vi "serialWrite.vi"(8 "error in (no error)":errorcluster, 10 "text":string, 11 "Python":T1) -> (0 "error out":errorcluster, 3 "Num loops":i32)   [LabVIEW 2020]
uses:
  PythonCtrl.ctl
  Processors.ctl
panel:
  out "appended array":i32[](array[numeric])
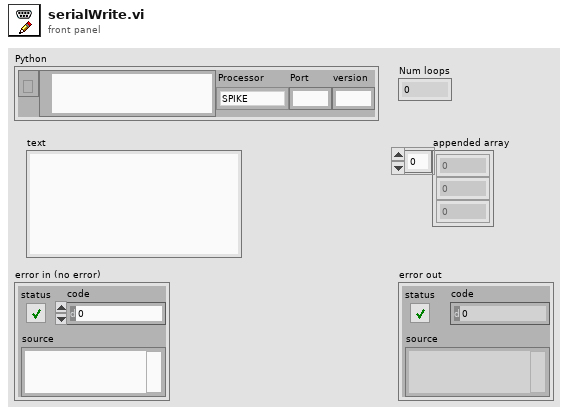
[diagram p1: front panel]
types:
  T1 = typedef "PythonCtrl.ctl" = cluster{"session":refnum<k35>, "PyPath":path, "Processor":T2, "Port":string, "version":string}
  T2 = typedef "Processors.ctl" = enum16{"SPIKE", "Pi", "Pi_ssh", "OpenMV", "Dunio"}
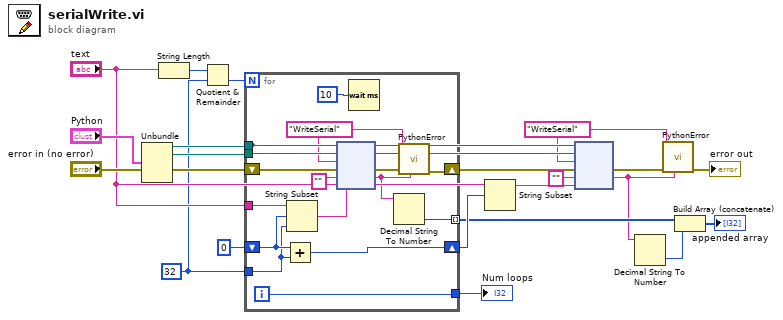
[diagram p0: block diagram]
diagram:
  w1 = "WriteSerial" ("function name")
  w11 = 32 ("length (rest)")
  n1 = Unbundle("Python") -> ("session"=w20:refnum<k35>, "PyPath"=w21:path)  [unwired: 3 out]
  n2 = String Length(string="text") -> (length=w12:i32)
  n3 = Quotient & Remainder(x=w12, y=w11) -> (floor(x/y)=w10:i32)  [unwired: 1 out]
  n4 = for {
    N: w10 -> [_]
    tunnel: "text" -> [w37]
    shift-right: [w35] -> w9
    shift-left: 0 -> [w36]
    tunnel: w11 -> [w34]
    tunnel: [w32] -> w18
    shift-right: [w26] -> w16
    shift-left: "error in (no error)" -> [w30]
    tunnel: w20 -> [w29]
    tunnel: w21 -> [w28]
    tunnel: [w24] -> w8 mode=indexing
    i -> [w32]
    w22 = "WriteSerial" ("function name")
    n5 = Add(x=w36, y=w34) -> (x+y=w35:i32)
    n6 = String Subset(string=w37, offset (0)=w36, length (rest)=w34) -> (substring=w31:string)
    n7 = node(w29, w28, w22, w30, "" ("function name"), w31) -> (w27:errorcluster, w23:string)  [unwired: 1 in, 3 out]
    n8 = Wait (ms)(milliseconds to wait=u32 10) -> ()  [unwired: 1 out]
    n9 = Decimal String To Number(string=w23) -> (number=w24:i32)  [unwired: 2 in, 1 out]
    n10 = call "PythonError.vi"("reply"=w23, "error in (no error)"=w27, "function name"=w22) -> ("error out"=w26:errorcluster)  [unwired: 8 in]
  }
  "Num loops" <- w18
  n11 = String Subset(string="text", offset (0)=w9) -> (substring=w17:string)  [unwired: 1 in]
  n12 = node(w20, w21, w1, w16, "" ("function name"), w17) -> (w6:errorcluster, w3:string)  [unwired: 1 in, 3 out]
  n13 = Decimal String To Number(string=w3) -> (number=w2:i32)  [unwired: 2 in, 1 out]
  n14 = call "PythonError.vi"("reply"=w3, "error in (no error)"=w6, "function name"=w1) -> ("error out"=→"error out":errorcluster)  [unwired: 8 in]
  n15 = Build Array (concatenate)(w8, w2) -> (→"appended array":i32[])
